vi "scan_updown.vi"() -> ()   [LabVIEW 2011, in "run.lvlib"]
doc: "I. Description:\nThis example demonstrates how to continuously output a waveform using an internal sample clock and a digital start trigger.\n\nII. Instructions for Running:\n1. Select the Physical Channel to correspond to where your signal is output on the DAQ device.\n2. Enter the Minimum and Maximum Voltage Ranges.\n3. Specify the Desired Frequency of the output Waveform\n4. Select the Digital Trigger Source.\n5. Specify the desired Trigger Edge.\n6. Enter the Waveform Information. See the documentation of the Waveform Buffer Generation SubVI for information on each parameter.\n\nIII. Block Diagram Steps:\n1. Create an Analog Output Voltage Task\n2.Call the DAQmx Timing (Use Waveform) VI which sets the sample clock rate based on the input waveform parameters, and set the sample mode to Continuous.\n3. Define the Triggering parameters: Source and Edge\n4. Write the waveform to the output buffer.\n5. Call the Start VI.\n6. Loop continuously until the user presses the Stop button. Check for errors every 100 ms using the Is Task Done? VI\n7. Call the Clear Task VI to clear the Task.\n8. Use the popup dialog box to display an error or warning if any.\n\nIV. I/O Connections Overview:\nMake sure your signal output terminal matches the Physical Channel I/O Control. Also, make sure your digital trigger terminal matches the Trigger Source Control. For further connection information, refer to your hardware reference manual."
uses:
  Hal/testing/run.lvlib
  <vilib>/Utility/error.llb/DialogType.ctl
  <vilib>/DAQmx/write.llb/DAQmx Write (Analog 1D Wfm NChan NSamp).vi
  <vilib>/DAQmx/create/channels.llb/DAQmx Create Channel (AO-Voltage-Basic).vi
  <vilib>/DAQmx/configure/timing.llb/DAQmx Timing (Use Waveform).vi
  <vilib>/DAQmx/miscellaneous.llb/DAQmx Fill In Error Info.vi
panel:
  in  "offset":dbl=2.0
  out "Resulting Frequency":dbl format="%.2f"
  in  "Cycles per Buffer":i32=15
  in  "Waveform Type":T1(ring)
  in  "Amplitude":dbl=0.5 caption="Amplitude Current" format="%0.2p"
  in  "Samples per Buffer":dbl=750.0
  in  "Desired Frequency":dbl=0.1 format="%.2f"
  out "Output Waveform":waveform(dbl)[](graph)
  in  "Physical Channels":tag="Ao8b/ao2"
  in  "Minimum Value":dbl=-10.0 format="%0.2f"
  in  "Maximum Value":dbl=10.0 format="%0.2f"
  in  "stop":bool
  # "For instructions, select Help>>Show Context Help"
  # "Channel Parameters"
  # "Timing Parameters"
  # "Waveform Information"
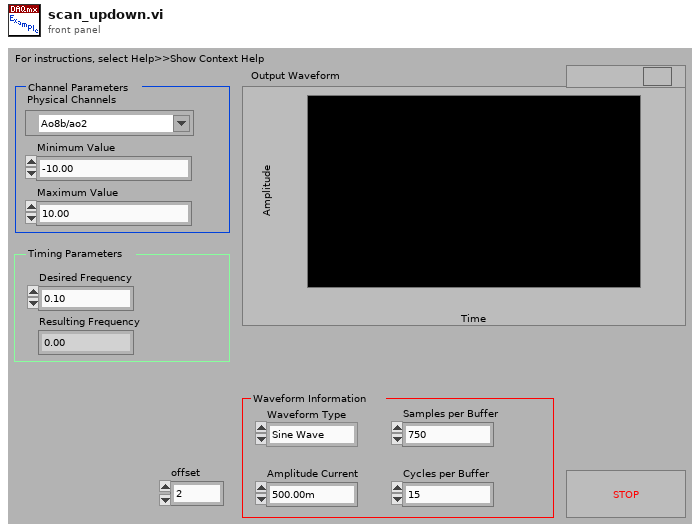
[diagram p1: front panel]
types:
  T1 = enum16{"Sine Wave", "Triangle Wave", "Square Wave", "Sawtooth Wave"}
  T2 = typedef "DialogType.ctl" = u16
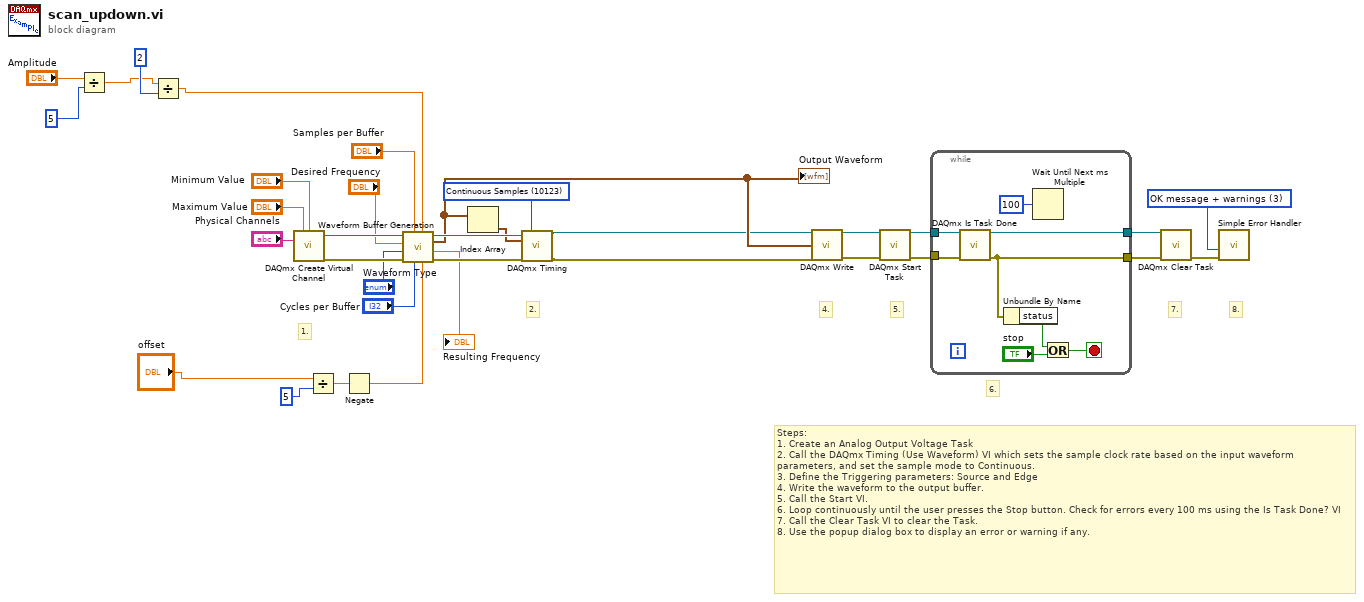
[diagram p0: block diagram]
diagram:
  w26 = T2 3 items=["no dialog", "OK message", "continue or stop message", "OK message + warnings", "continue/stop + warnings"] ("type of dialog (OK msg:1)")
  w33 = 10123 items=["Finite Samples"=10178, "Continuous Samples"=10123] ("sample mode")
  # "8."
  # "6."
  # "7."
  # "Steps: \n1. Create an Analog Output Voltage Task\n2. Call the DAQmx Timing (Use Waveform) VI which sets the sample clock rate based on the input waveform parameters, and set the sample mode to Continuous.\n3. Define the Triggering parameters: Source and Edge\n4. Write the waveform to the output buffer.\n5. Call the Start VI.\n6. Loop continuously until the user presses the Stop button. Check for errors every 100 ms using the Is Task Done? VI\n7. Call the Clear Task VI to clear the Task.\n8. Use the popup dialog box to display an error or warning if any."
  # "5."
  # "4."
  # "2."
  # "1."
  n1 = Divide(x="Amplitude", y=5) -> (x/y=w3:dbl)
  n2 = Divide(x=w3, y=2) -> (x/y=w5:dbl)
  n3 = call-poly <vilib>:"DAQmx Create Virtual Channel.vi"("maximum value"="Maximum Value", "minimum value"="Minimum Value", "physical channels"="Physical Channels") -> ("task out"=w20:refnum<k21>, "error out"=w22:errorcluster)  [unwired: 11 in]
  n4 = Divide(x="offset", y=5) -> (x/y=w7:dbl)
  n5 = Negate(x=w7) -> (-x=w6:dbl)
  n6 = call "Waveform Buffer Generation.vi"("offset"=w6, "Amplitude"=w5, "Cycles per Buffer"="Cycles per Buffer", "Samples per Buffer"="Samples per Buffer", "error in (no error)"=w22, "Waveform Type"="Waveform Type", "Desired Frequency"="Desired Frequency", "task/channels in"=w20) -> ("error out"=w21:errorcluster, "Resulting Frequency"=→"Resulting Frequency":dbl, "Waveform"=w13:waveform(dbl)[], "task out"=w15:refnum<k21>)
  "Output Waveform" <- w13
  n7 = Index Array(array=w13) -> (element=w12:waveform(dbl))  [unwired: 1 in]
  n8 = call-poly <vilib>:"DAQmx Timing.vi"("task/channels in"=w15, "sample mode"=w33, "waveform"=w12, "error in"=w21) -> ("task out"=w11:refnum<k21>, "error out"=w10:errorcluster)  [unwired: 10 in]
  n9 = call-poly <vilib>:"DAQmx Write.vi"("task/channels in"=w11, "data"=w13, "error in"=w10) -> ("task out"=w30:refnum<k21>, "error out"=w29:errorcluster)  [unwired: 10 in, 1 out]
  n10 = call <vilib>:"DAQmx Start Task.vi"("task/channels in"=w30, "error in"=w29) -> ("task out"=w34:refnum<k21>, "error out"=w28:errorcluster)  [unwired: 12 in]
  n11 = while {
    tunnel: w34 -> [w38]
    tunnel: [w35] -> w24
    tunnel: w28 -> [w37]
    tunnel: [w36] -> w23
    stop <- w42 stop-if-true
    n12 = call <vilib>:"DAQmx Is Task Done.vi"("task/channels in"=w38, "error in"=w37) -> ("task out"=w35:refnum<k21>, "error out"=w36:errorcluster)  [unwired: 11 in, 1 out]
    n13 = Unbundle By Name(w36) -> ("status"=w40:bool)
    n14 = Wait Until Next ms Multiple(millisecond multiple=u32 100) -> ()  [unwired: 1 out]
    n15 = Or(x=w40, y="stop") -> (x .or. y?=w42:bool)
  }
  n16 = call <vilib>:"DAQmx Clear Task.vi"("task in"=w24, "error in"=w23) -> ("error out"=w25:errorcluster)  [unwired: 13 in]
  n17 = call <vilib>:"Simple Error Handler.vi"("type of dialog (OK msg:1)"=w26, "error in (no error)"=w25) -> ()  [unwired: 3 in, 5 out]
